vi "Read Setpoint Temperature.vi"(8 "error in (no error)":errorcluster, 11 "Thermal Chamber Response Simlator In":refnum<class "Thermal Chamber Response Simlator.lvclass">) -> (0 "error out":errorcluster, 2 "Setpoint Temperature [degC]":dbl, 3 "Thermal Chamber Response Simlator Out":refnum<class "Thermal Chamber Response Simlator.lvclass">)   [LabVIEW 2020, in "Thermal Chamber Response Simlator.lvclass"]
uses:
  Thermal Chamber Response Simlator.lvclass
  Thermal Chamber Response Simlator.lvclass/Thermal Chamber Response Simlator.ctl
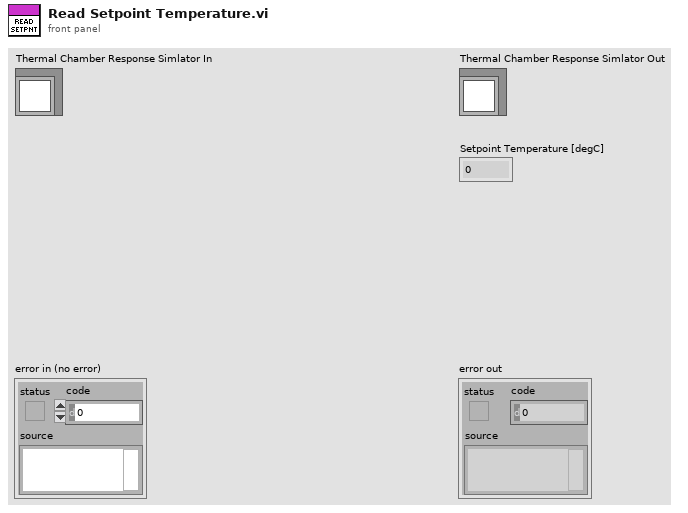
[diagram p1: front panel]
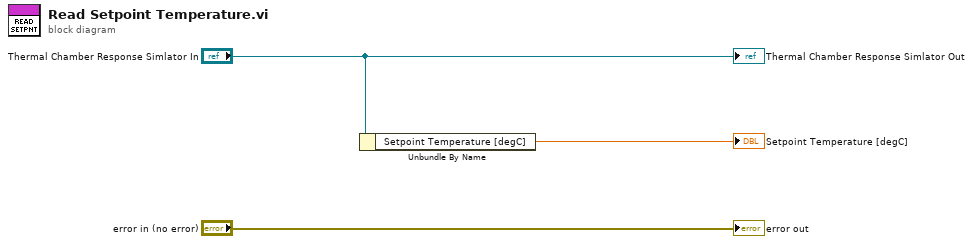
[diagram p0: block diagram]
diagram:
  n1 = Unbundle By Name("Thermal Chamber Response Simlator In") -> ("Setpoint Temperature [degC]"=→"Setpoint Temperature [degC]":dbl)
  "error out" <- "error in (no error)"
  "Thermal Chamber Response Simlator Out" <- "Thermal Chamber Response Simlator In"
